vi "Throttle.vi"(10 "Throttle (ms)":u32) -> (2 "Past Throttle":bool)   [LabVIEW 2014, in "Robot Actor Framework.lvlib" / "Utilities.lvlib"]
uses:
  Utilities.lvlib
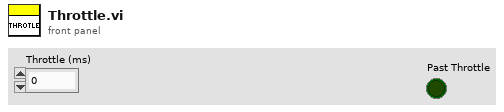
[diagram p1: front panel]
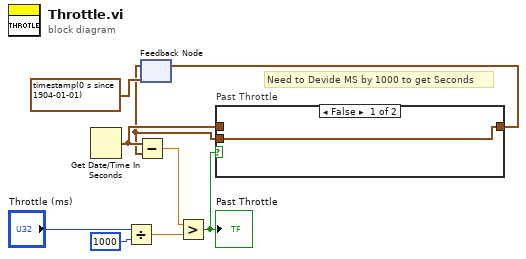
[diagram p0: block diagram]
diagram:
  # "Need to Devide MS by 1000 to get Seconds"
  n1 = Get Date/Time In Seconds() -> (seconds since 1Jan1904=w3:timestamp)
  n2 = Divide(x="Throttle (ms)", y=u32 1000) -> (x/y=w5:dbl)
  n3 = feedback #1(timestamp(0 s since 1904-01-01)) -> (w1:timestamp)
  n4 = Subtract(x=w3, y=w1) -> (x-y=w6:dbl)
  n5 = Greater?(x=w6, y=w5) -> (0:w4:bool)
  "Past Throttle" <- w4
  n6 = case "Past Throttle" shown="False" w4 {
    tunnel: w3 -> [_ w11]
    tunnel: [w10 w11] -> w2
    tunnel: w1 -> [w10 _]
    frame False {
    }
    frame True {
    }
  }
  n7 = feedback-in #1(w2) -> ()
